vi "Destroy.vi"(11 "jettl Event Actor in":refnum<class "jettl Event Actor.lvclass">) -> ()   [LabVIEW 2021, in "jettl.lvlib" / "jettl Event Actor.lvlib" / "jettl Event Actor.lvclass"]
uses:
  jettl Event Actor.lvclass
  jettl Event Actor.lvclass/jettl Event Actor.ctl
  Actor/Msgs/Event Last Ack/Event Last Ack Msg/Event Last Ack Msg.lvclass
  C:/git/jettl/src/jettl/jettl Event Actor/jettl Event Actor/jettl Event Actor.lvclass
  C:/git/jettl/src/Actor/Event Actor/Event Actor.lvclass
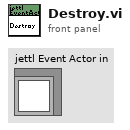
[diagram p1: front panel]
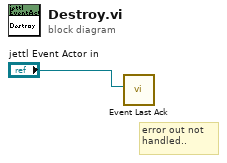
[diagram p0: block diagram]
diagram:
  # "error out not handled.."
  n1 = call "Event Last Ack.vi"("Event Actor"="jettl Event Actor in") -> ()  [unwired: 10 in, 1 out]
